vi "Import Payload File.vi"(8 "error in (no error)":errorcluster, 10 "payload file path":path, 11 "custom device ref in":T1 format="%.0x") -> (0 "error out":errorcluster, 3 "custom device ref out out":T1 format="%.0x")   [LabVIEW 2020, in "AIM ARINC 664 Scripting.lvlib"]
uses:
  AIM ARINC 664 Scripting.lvlib
  <vilib>/NI VeriStand/Custom Device API/Custom Device Item Ref.ctl
  <vilib>/NI VeriStand/Custom Device API/Custom Device API.lvlib
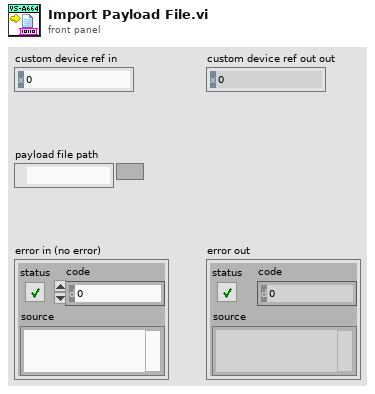
[diagram p1: front panel]
types:
  T1 = typedef "Custom Device API.lvlib/Custom Device Item Ref.ctl" = u64
  T2 = typedef "Payload Map.ctl" = map{string, T3}
  T3 = typedef "Payload Record Type.ctl" = cluster{"Data":u8[], "Type of Frame":T4}
  T4 = typedef "Type of Payload.ctl" = u16
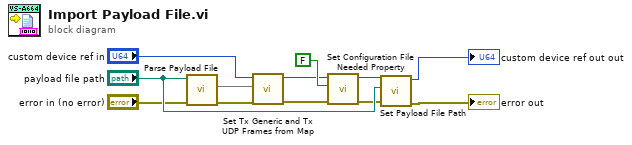
[diagram p0: block diagram]
diagram:
  n1 = call "Parse Payload File.vi"("error in"="error in (no error)", "frame array path in"="payload file path") -> ("error out"=w2:errorcluster, "Map"=w3:T2)  [unwired: 7 in, 1 out]
  n2 = call "Set Tx Generic and Tx UDP Frames from Map.vi"("error in"=w2, "payload map"=w3, "custom device ref"="custom device ref in") -> ("error out"=w9:errorcluster, "custom device ref out"=w4:T1)  [unwired: 7 in]
  n3 = call "Set Configuration File Needed Property.vi"("error in"=w9, "needed?"=FALSE, "custom device ref in"=w4) -> ("error out"=w7:errorcluster, "custom device ref out"=w8:T1)  [unwired: 7 in]
  n4 = call "Set Payload File Path.vi"("error in"=w7, "frame array file path"="payload file path", "custom device ref in"=w8) -> ("error out"=→"error out":errorcluster, "custom device ref out out"=→"custom device ref out out":T1)  [unwired: 7 in]
